vi "Update UI.vi"(8 "error in (no error)":errorcluster, 10 "DataExchange":T1, 11 "Laser Oxxius Controller in":refnum<class "LaserController.lvclass">) -> (0 "error out":errorcluster, 3 "Laser Oxxius Controller out":refnum<class "LaserController.lvclass">)   [LabVIEW 2020, in "LaserController.lvlib" / "LaserController.lvclass"]
uses:
  LaserController.lvclass
  Model/Hardware Abstraction Layer/Component/Device/Device/DataExchange.ctl
  LaserController.lvclass/LaserController.ctl
  Interface/DataListener/DataListener.lvclass
panel:
  out "error out 2":errorcluster
  in  "event data":cluster{"Label":string, "Value":dbl}
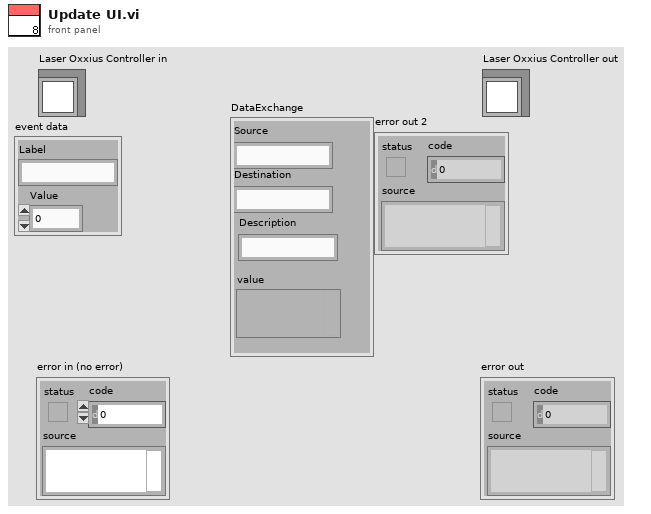
[diagram p1: front panel]
types:
  T1 = typedef "DataListener.lvclass/DataExchange.ctl" = cluster{"Source":string, "Destination":string, "Description":string, "value":variant}
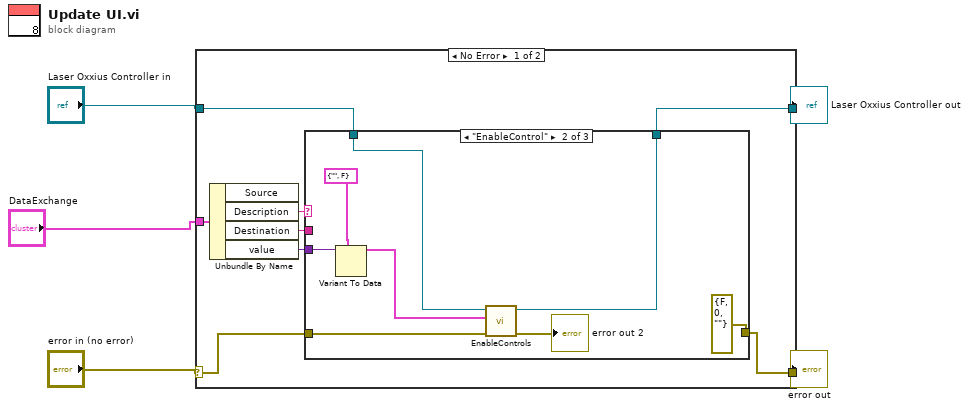
[diagram p0: block diagram]
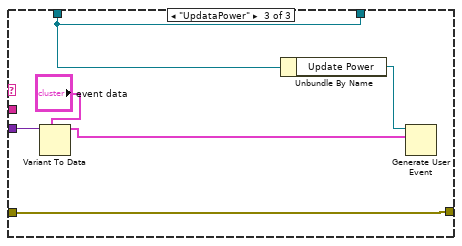
[diagram p3: hidden frame]
diagram:
  n1 = case shown="No Error" "error in (no error)" {
    selector: "error in (no error)" -> [w7 w31]
    tunnel: [w6 w31] -> w4
    tunnel: [w8 w30] -> w5
    tunnel: "Laser Oxxius Controller in" -> [w9 w30]
    tunnel: "DataExchange" -> [w13 _]
    frame No Error {
      n2 = Unbundle By Name(w13) -> ("Description"=w10:string, "Destination"=w11:string, "value"=w12:variant)  [unwired: 1 out]
      n3 = case shown="\"EnableControl\"" w10 {
        tunnel: w12 -> [_ w23 w29]
        tunnel: w11 -> [_ _ _]
        tunnel: w9 -> [w15 w21 w25]
        tunnel: [w15 w20 w25] -> w8
        tunnel: [w14 errorcluster {"status"=FALSE, "code"=0, "source"=""} ("error IO") w24] -> w6
        tunnel: w7 -> [w14 w22 w24]
        frame "False", Default {
        }
        frame "EnableControl" {
          n4 = Variant To Data(type=cluster{"Label":string, "Visable?":bool} {"Label"="", "Visable?"=FALSE} ("event data"), Variant=w23) -> (data=w16:cluster{"Label":string, "Visable?":bool})  [unwired: 1 in, 1 out]
          n5 = call-dynamic "EnableControls.vi"("error in (no error)"=w22, "event data"=w16, "OxxiusLaserController in"=w21) -> ("error out"=→"error out 2":errorcluster, "OxxiusLaserController out"=w20:refnum<class "LaserController.lvclass">)  [unwired: 7 in]
        }
        frame "UpdataPower" {
          n6 = Variant To Data(type="event data", Variant=w29) -> (data=w26:cluster{"Label":string, "Value":dbl})  [unwired: 1 in, 1 out]
          n7 = Unbundle By Name(w25) -> ("Update Power"=w28:refnum<user-event>)
          n8 = Generate User Event(user event=w28, event data cluster=w26) -> ()  [unwired: 2 in, 2 out]
        }
      }
    }
    frame Error {
    }
  }
  "error out" <- w4
  "Laser Oxxius Controller out" <- w5
